vi "EdwardsPumpRead.vi"(1 "Pump Address":refnum<visa-resource-name>) -> (0 "Gauge 1 mBar":dbl format="%#.1e")   [LabVIEW 2025]
doc: "Author: Scott Hannahs <sth@magnet.fsu.edu>\n\nThis software is licensed for use under the “MIT License\"\nCopyright (c) 2025 Scott Hannahs, sth@sth@magnet.sthnet.net\n\nPermission is hereby granted, free of charge, to any person obtaining a copy of this software and associated documentation files (the \"Software\"), to deal in the Software without restriction, including without limitation the rights to use, copy, modify, merge, publish, distribute, sublicense, and/or sell copies of the Software, and to permit persons to whom the Software is furnished to do so, subject to the following conditions: The above copyright notice and this permission notice shall be included in all copies or substantial portions of the Software.\n\nTHE SOFTWARE IS PROVIDED \"AS IS\", WITHOUT WARRANTY OF ANY KIND, EXPRESS OR IMPLIED, INCLUDING BUT NOT LIMITED TO THE WARRANTIES OF MERCHANTABILITY, FITNESS FOR A PARTICULAR PURPOSE AND NONINFRINGEMENT. IN NO EVENT SHALL THE AUTHORS OR COPYRIGHT HOLDERS BE LIABLE FOR ANY CLAIM, DAMAGES OR OTHER LIABILITY, WHETHER IN AN ACTION OF CONTRACT, TORT OR OTHERWISE, ARISING FROM, OUT OF OR IN CONNECTION WITH THE SOFTWARE OR THE USE OR OTHER DEALINGS IN THE SOFTWARE."
panel:
  in  "Tab Control":enum32{"Gauge 1", "Gauge 2"}(tab)
  out "Gauge 2 mBar":dbl format="%#.1e"
  out "error out 2":errorcluster
  in  "Boolean":bool
  out "Pressure out":variant
  out "error out":errorcluster
  in  "stop":bool
  # "GAUGES:"
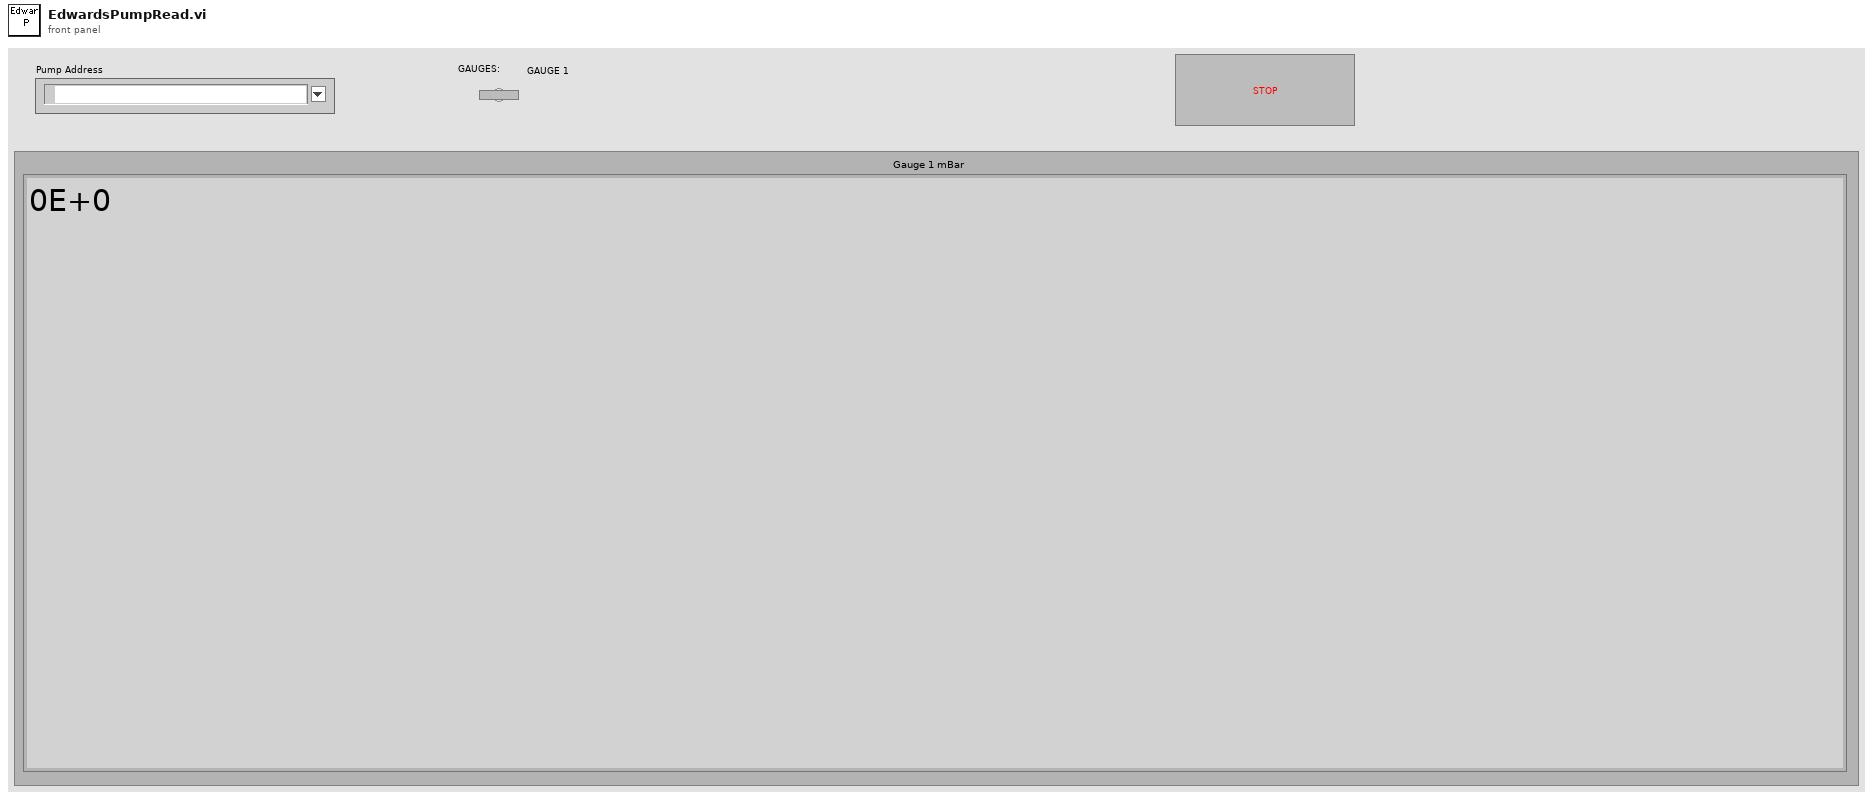
[diagram p1: front panel]
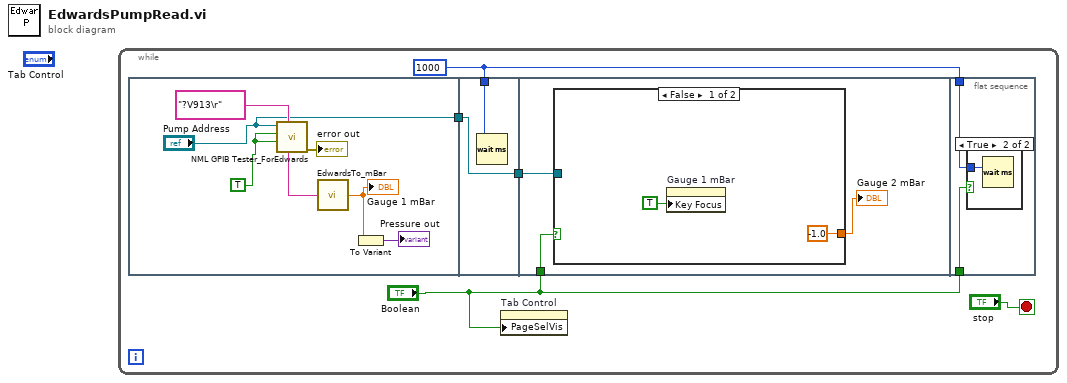
[diagram p0: block diagram]
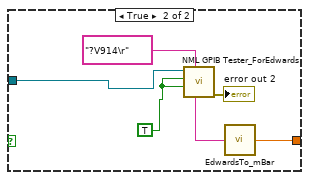
[diagram p2: hidden frame]
diagram:
  n1 = while {
    stop <- "stop" stop-if-true
    w4 = u32 1000 ("milliseconds to wait")
    n2 = flat-sequence {
      tunnel: ["Pump Address"] -> w3
      tunnel: w4 -> [w14]
      tunnel: w3 -> [w13]
      tunnel: [w13] -> w2
      tunnel: "Boolean" -> [w17]
      tunnel: w2 -> [w16]
      tunnel: "Boolean" -> [w27]
      tunnel: w4 -> [w26]
      frame #0 {
        w11 = TRUE ("Write")
        n3 = call "NML GPIB Tester_ForEdwards.vi"(5:"?V913\r", "Read"=w11, "Write"=w11, "VISA resource name"="Pump Address") -> ("error out"=→"error out":errorcluster, 4:w8:string)  [unwired: 4 in]
        n4 = call "EdwardsTo_mBar.vi"("Input"=w8) -> ("mBar"=w7:dbl)
        "Gauge 1 mBar" <- w7
        n5 = To Variant(anything=w7) -> (Variant=→"Pressure out":variant)
      }
      frame #1 {
        n6 = Wait (ms)(milliseconds to wait=w14) -> ()  [unwired: 1 out]
      }
      frame #2 {
        n7 = case shown="False" w17 {
          tunnel: w16 -> [_ w21]
          tunnel: [-1.0 ("mBar") w20] -> w15
          frame False {
            n8 = property on="Gauge 1 mBar" class="DigNum (strict)"("Key Focus"=TRUE) -> ()  [unwired: 2 in, 2 out]
          }
          frame True {
            w24 = TRUE ("Write")
            n9 = call "NML GPIB Tester_ForEdwards.vi"(5:"?V914\r", "Read"=w24, "Write"=w24, "VISA resource name"=w21) -> ("error out"=→"error out 2":errorcluster, 4:w22:string)  [unwired: 4 in]
            n10 = call "EdwardsTo_mBar.vi"("Input"=w22) -> ("mBar"=w20:dbl)
          }
        }
        "Gauge 2 mBar" <- w15
      }
      frame #3 {
        n11 = case shown="True" w27 {
          tunnel: w26 -> [_ w28]
          frame False {
          }
          frame True {
            n12 = Wait (ms)(milliseconds to wait=w28) -> ()  [unwired: 1 out]
          }
        }
      }
    }
    n13 = property on="Tab Control" class="TabCtl (strict)"("PageSelVis"="Boolean") -> ()  [unwired: 2 in, 2 out]
  }
